vi "LoadSTL.vi"(11 "STL Path":path) -> (1 "NumFaces":u32, 2 "Title":string, 3 "Triangles":T1[](array[typedef]))   [LabVIEW 2014]
uses:
  TypeDefs/TriangleFace.ctl
  TypeDefs/Point3D.ctl
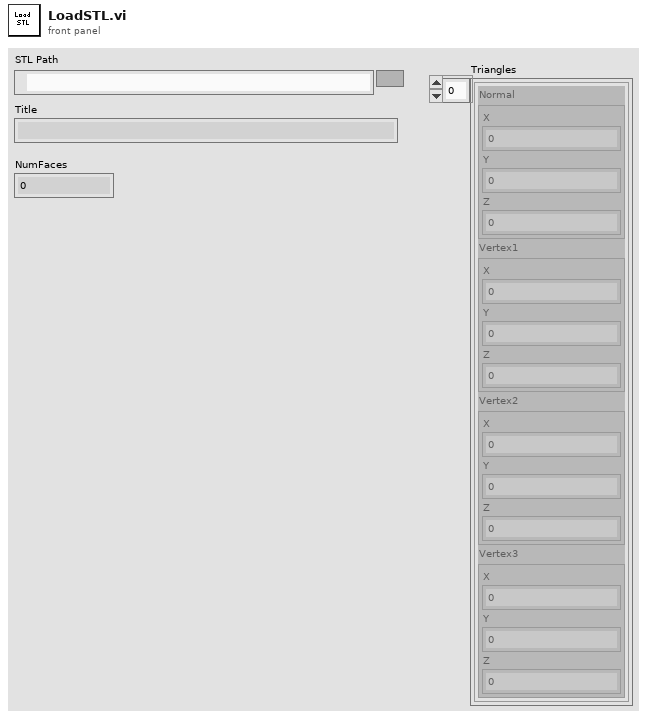
[diagram p1: front panel]
types:
  T1 = typedef "TriangleFace.ctl" = cluster{"Normal":T2, "Vertex1":T2, "Vertex2":T2, "Vertex3":T2}
  T2 = typedef "Point3D.ctl" = cluster{"X":sgl, "Y":sgl, "Z":sgl}
  T3 = enum16{"big-endian, network order", "native, host order", "little-endian"}
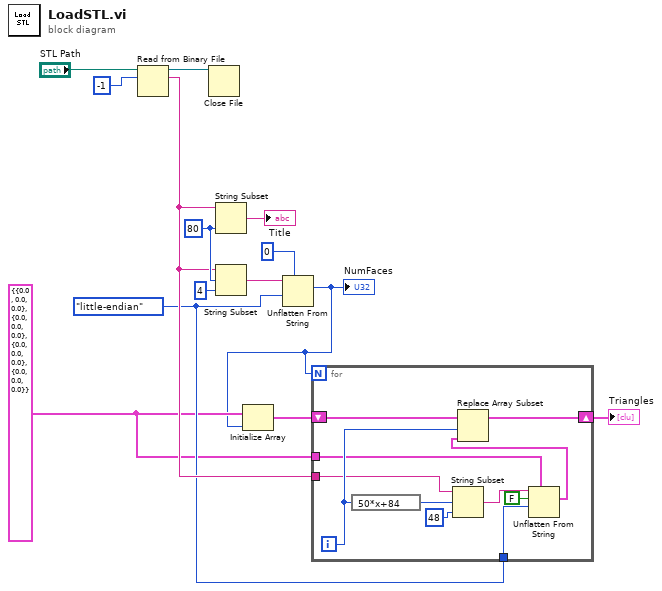
[diagram p0: block diagram]
diagram:
  w3 = T1 {"Normal"={"X"=0.0, "Y"=0.0, "Z"=0.0}, "Vertex1"={"X"=0.0, "Y"=0.0, "Z"=0.0}, "Vertex2"={"X"=0.0, "Y"=0.0, "Z"=0.0}, "Vertex3"={"X"=0.0, "Y"=0.0, "Z"=0.0}} ("TriangleFace")
  w4 = T3."little-endian" ("byte order (0:big-endian, network order)")
  w10 = 80 ("length (rest)")
  n1 = Read from Binary File(10:-1 ("count (1)"), 11:"STL Path") -> (2:w5:string, 3:w13:refnum<file>)  [unwired: 4 in, 2 out]
  n2 = Close File(refnum=w13) -> ()  [unwired: 1 in, 2 out]
  n3 = String Subset(string=w5, length (rest)=w10) -> (substring=→"Title":string)  [unwired: 1 in]
  n4 = String Subset(string=w5, offset (0)=w10, length (rest)=4 ("length (rest)")) -> (substring=w8:string)
  n5 = Unflatten From String(type=u32 0, binary string=w8, byte order (0:big-endian, network order)=w4) -> (value=w1:u32)  [unwired: 2 in, 2 out]
  "NumFaces" <- w1
  n6 = Initialize Array(w3, w1) -> (w6:T1[])
  n7 = for {
    N: w1 -> [_]
    tunnel: w5 -> [w21]
    tunnel: w4 -> [w19]
    tunnel: w3 -> [w17]
    shift-right: [w15] -> w2
    shift-left: w6 -> [w25]
    i -> [w24]
    n8 = expression code="50*x+84"(w24) -> (w23:i32)
    n9 = String Subset(string=w21, offset (0)=w23, length (rest)=48 ("length (rest)")) -> (substring=w20:string)
    n10 = Unflatten From String(type=w17, binary string=w20, data includes array or string size? (T)=FALSE, byte order (0:big-endian, network order)=w19) -> (value=w16:T1)  [unwired: 1 in, 2 out]
    n11 = Replace Array Subset(array=w25, new element=w16, index=w24) -> (w15:T1[])
  }
  "Triangles" <- w2
